vi "R1pHControl.vi"(8 "error constant":errorcluster, 11 "LabVIEW Web Service":refnum<class "Web Service.lvclass">) -> ()   [LabVIEW 2016]
uses:
  <vilib>/wsapi/Web Service.lvclass
  Controls/pH_SetParams Standard.ctl
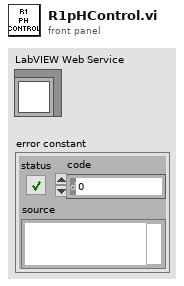
[diagram p1: front panel]
types:
  T1 = cluster{"Media Pump":bool, "Water Pump":bool, "Gas Pump":bool, "Effluent Pump":bool}
  T2 = typedef "pH_SetParams Standard.ctl" = cluster{"Set Point":dbl, "Tolerance":dbl, "Pump Time On, secs":dbl}
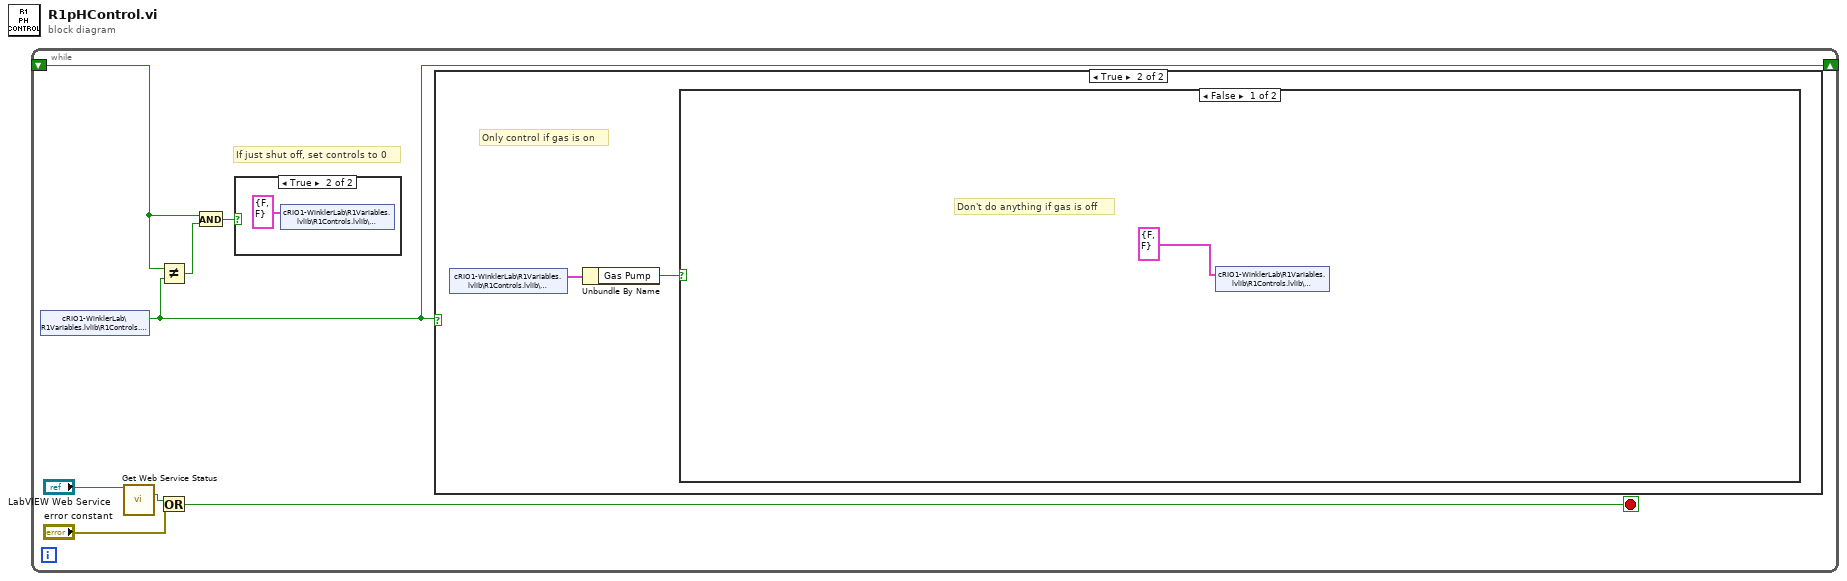
[diagram p0: block diagram]
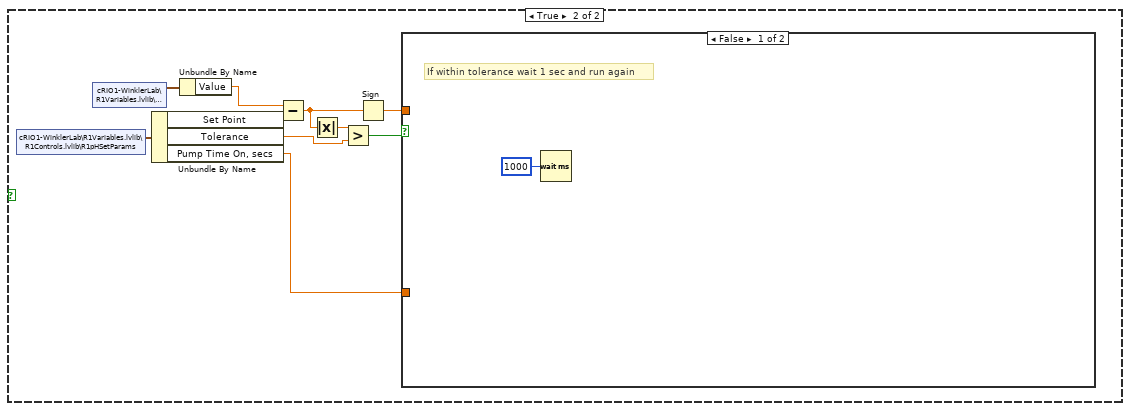
[diagram p4: hidden frame]
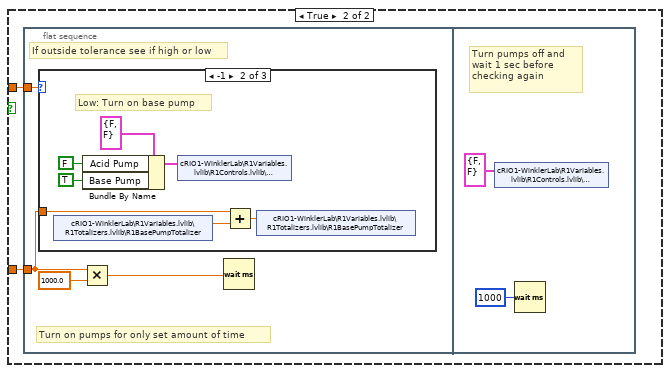
[diagram p5: hidden frame]
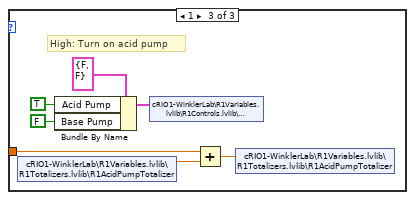
[diagram p7: hidden frame]
diagram:
  n1 = while {
    shift-right: [w3] -> _
    shift-left: _ -> [w2]
    stop <- w5 stop-if-true
    # "If just shut off, set controls to 0"
    n2 = shared-variable "cRIO1-WinklerLab\\R1Variables.lvlib\\R1Controls.lvlib\\R1pHSwitch"() -> (w3:bool)  [unwired: 1 in, 1 out]
    n3 = call <vilib>:"Get Web Service Status.vi"("LabVIEW Web Service"="LabVIEW Web Service") -> ("service stopping?"=w8:bool)  [unwired: 12 in, 2 out]
    n4 = Not Equal?(x=w2, y=w3) -> (x != y?=w4:bool)
    n5 = Or(x=w8, y="error constant") -> (x .or. y?=w5:bool)
    n6 = And(x=w2, y=w4) -> (x .and. y?=w1:bool)
    n7 = case shown="True" w1 {
      frame False {
      }
      frame True {
        n8 = shared-variable "cRIO1-WinklerLab\\R1Variables.lvlib\\R1Controls.lvlib\\R1pHManual"(cluster{"Acid Pump":bool, "Base Pump":bool} {"Acid Pump"=FALSE, "Base Pump"=FALSE} ("R1pHManual")) -> ()  [unwired: 1 in, 1 out]
      }
    }
    n9 = case shown="True" w3 {
      frame False {
        # "Don't do anything if control is off"
      }
      frame True {
        # "Only control if gas is on"
        n10 = shared-variable "cRIO1-WinklerLab\\R1Variables.lvlib\\R1Controls.lvlib\\R1SBRManual"() -> (w11:T1)  [unwired: 1 in, 1 out]
        n11 = Unbundle By Name(w11) -> ("Gas Pump"=w10:bool)
        n12 = case shown="False" w10 {
          frame False {
            # "Don't do anything if gas is off"
            n13 = shared-variable "cRIO1-WinklerLab\\R1Variables.lvlib\\R1Controls.lvlib\\R1pHManual"(cluster{"Acid Pump":bool, "Base Pump":bool} {"Acid Pump"=FALSE, "Base Pump"=FALSE} ("R1pHManual")) -> ()  [unwired: 1 in, 1 out]
          }
          frame True {
            n14 = shared-variable "cRIO1-WinklerLab\\R1Variables.lvlib\\R1Controls.lvlib\\R1pHSetParams"() -> (w21:T2)  [unwired: 1 in, 1 out]
            n15 = shared-variable "cRIO1-WinklerLab\\R1Variables.lvlib\\R1Signals.lvlib\\R1pH"() -> (w22:cluster{"Signal":dbl, "Value":dbl})  [unwired: 1 in, 1 out]
            n16 = Unbundle By Name(w21) -> ("Set Point"=w19:dbl, "Tolerance"=w17:dbl, "Pump Time On, secs"=w13:dbl)
            n17 = Unbundle By Name(w22) -> ("Value"=w20:dbl)
            n18 = Subtract(x=w20, y=w19) -> (x-y=w15:dbl)
            n19 = Absolute Value(x=w15) -> (abs(x)=w18:dbl)
            n20 = Greater?(x=w18, y=w17) -> (0:w16:bool)
            n21 = Sign(1:w15) -> (0:w14:dbl)
            n22 = case shown="False" w16 {
              tunnel: w14 -> [_ w25]
              tunnel: w13 -> [_ w24]
              frame False {
                # "If within tolerance wait 1 sec and run again"
                n23 = Wait (ms)(milliseconds to wait=u32 1000) -> ()  [unwired: 1 out]
              }
              frame True {
                n24 = flat-sequence {
                  tunnel: w25 -> [w29]
                  tunnel: w24 -> [w26]
                  frame #0 {
                    # "Turn on pumps for only set amount of time"
                    # "If outside tolerance see if high or low"
                    n25 = case shown="-1" w29 {
                      tunnel: w26 -> [_ w30 w39]
                      frame 0, Default {
                        # "Unless tolerance is 0 this code\nshouldn't be accesible"
                      }
                      frame -1 {
                        # "Low: Turn on base pump"
                        n26 = shared-variable "cRIO1-WinklerLab\\R1Variables.lvlib\\R1Totalizers.lvlib\\R1BasePumpTotalizer"() -> (w32:dbl)  [unwired: 1 in, 1 out]
                        n27 = Bundle By Name(cluster=cluster{"Acid Pump":bool, "Base Pump":bool} {"Acid Pump"=FALSE, "Base Pump"=FALSE} ("R1pHManual"), "Acid Pump"=FALSE, "Base Pump"=TRUE) -> (w35:cluster{"Acid Pump":bool, "Base Pump":bool})
                        n28 = shared-variable "cRIO1-WinklerLab\\R1Variables.lvlib\\R1Controls.lvlib\\R1pHManual"(w35) -> ()  [unwired: 1 in, 1 out]
                        n29 = Add(x=w30, y=w32) -> (x+y=w31:dbl)
                        n30 = shared-variable "cRIO1-WinklerLab\\R1Variables.lvlib\\R1Totalizers.lvlib\\R1BasePumpTotalizer"(w31) -> ()  [unwired: 1 in, 1 out]
                      }
                      frame 1 {
                        # "High: Turn on acid pump"
                        n31 = shared-variable "cRIO1-WinklerLab\\R1Variables.lvlib\\R1Totalizers.lvlib\\R1AcidPumpTotalizer"() -> (w38:dbl)  [unwired: 1 in, 1 out]
                        n32 = Bundle By Name(cluster=cluster{"Acid Pump":bool, "Base Pump":bool} {"Acid Pump"=FALSE, "Base Pump"=FALSE} ("R1pHManual"), "Acid Pump"=TRUE, "Base Pump"=FALSE) -> (w42:cluster{"Acid Pump":bool, "Base Pump":bool})
                        n33 = shared-variable "cRIO1-WinklerLab\\R1Variables.lvlib\\R1Controls.lvlib\\R1pHManual"(w42) -> ()  [unwired: 1 in, 1 out]
                        n34 = Add(x=w39, y=w38) -> (x+y=w37:dbl)
                        n35 = shared-variable "cRIO1-WinklerLab\\R1Variables.lvlib\\R1Totalizers.lvlib\\R1AcidPumpTotalizer"(w37) -> ()  [unwired: 1 in, 1 out]
                      }
                    }
                    n36 = Multiply(x=w26, y=1000.0) -> (x*y=w27:dbl)
                    n37 = Wait (ms)(milliseconds to wait=w27) -> ()  [unwired: 1 out]
                  }
                  frame #1 {
                    # "Turn pumps off and \nwait 1 sec before\nchecking again"
                    n38 = shared-variable "cRIO1-WinklerLab\\R1Variables.lvlib\\R1Controls.lvlib\\R1pHManual"(cluster{"Acid Pump":bool, "Base Pump":bool} {"Acid Pump"=FALSE, "Base Pump"=FALSE} ("R1pHManual")) -> ()  [unwired: 1 in, 1 out]
                    n39 = Wait (ms)(milliseconds to wait=u32 1000) -> ()  [unwired: 1 out]
                  }
                }
              }
            }
          }
        }
      }
    }
  }
